vi "test Get LabVIEW Version.vi"(8 "Error In":errorcluster) -> (0 "Error Out":errorcluster)   [LabVIEW 2015, in "unit tests.lvlib"]
uses:
  unit tests.lvlib
  <vilib>/addons/_JKI Toolkits/Caraya/classes/Assert/Assert Equal Value_Variant.vi
  <vilib>/addons/_JKI Toolkits/Caraya/classes/Test/Test.lvclass
  LV Project Version Check.lvlib
  <vilib>/addons/_JKI Toolkits/Caraya/classes/Assert/Assert.lvclass
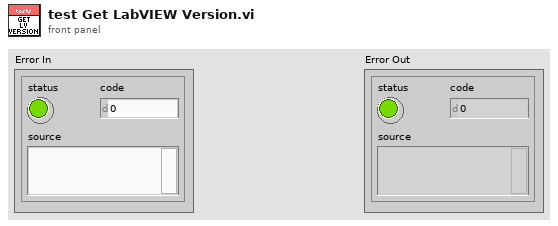
[diagram p1: front panel]
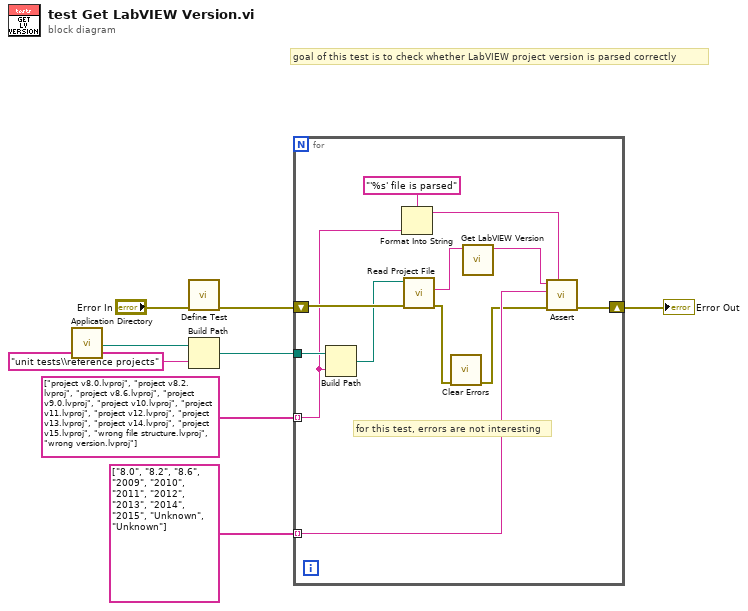
[diagram p0: block diagram]
diagram:
  # "goal of this test is to check whether LabVIEW project version is parsed correctly"
  n1 = call <vilib>:"Application Directory.vi"() -> ("Application Directory"=w7:path)
  n2 = call <vilib>:"Define Test.vi"("error in (no error)"="Error In") -> ("error out"=w5:errorcluster)  [unwired: 10 in]
  n3 = Build Path(base path=w7, name or relative path="unit tests\\reference projects") -> (appended path=w3:path)
  n4 = for {
    shift-right: [w16] -> w4
    shift-left: w5 -> [w19]
    tunnel: w3 -> [w20]
    tunnel: string[] ["project v8.0.lvproj", "project v8.2.lvproj", "project v8.6.lvproj", "project v9.0.lvproj", "project v10.lvproj", "project v11.lvproj", "project v12.lvproj", "project v13.lvproj", "project v14.lvproj", "project v15.lvproj", "wrong file structure.lvproj", "wrong version.lvproj"] ("filenames") -> [w12] mode=indexing
    tunnel: string[] ["8.0", "8.2", "8.6", "2009", "2010", "2011", "2012", "2013", "2014", "2015", "Unknown", "Unknown"] ("filenames") -> [w13] mode=indexing
    # "for this test, errors are not interesting"
    n5 = Build Path(base path=w20, name or relative path=w12) -> (appended path=w18:path)
    n6 = Format Into String(format string="'%s' file is parsed", w12) -> (resulting string=w10:string)  [unwired: 2 in, 1 out]
    n7 = call "Read Project File.vi"("Error In"=w19, "path to XML document"=w18) -> ("Error Out"=w15:errorcluster, "Project Version out"=w17:string)  [unwired: 7 in, 1 out]
    n8 = call <vilib>:"Clear Errors.vi"("error in (no error)"=w15) -> ("error out"=w9:errorcluster)  [unwired: 5 in, 1 out]
    n9 = call "Get LabVIEW Version.vi"("Project Version String"=w17) -> ("Version (string) out"=w14:string)  [unwired: 9 in, 1 out]
    n10 = call-poly <vilib>:"Assert.vi"("Label"=w10, "error in (no error)"=w9, "Y"=w13, "X"=w14) -> ("error out"=w16:errorcluster)  [unwired: 7 in]
  }
  "Error Out" <- w4
